vi "TCP Recieve Message.vi"(6 "Close on error":bool, 7 "Magic":u32=3737844653 format="%x", 8 "Error In":errorcluster, 11 "connection ID":refnum<k5>) -> (0 "Error Out":errorcluster, 1 "Valid":bool, 2 "Response":string, 3 "connection ID out":refnum<k5>)   [LabVIEW 2019]
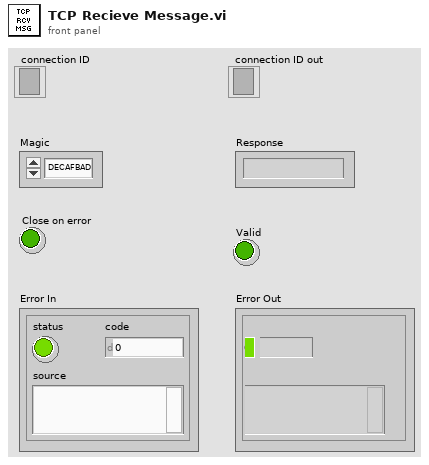
[diagram p1: front panel]
types:
  T1 = enum16{"big-endian, network order", "native, host order", "little-endian"}
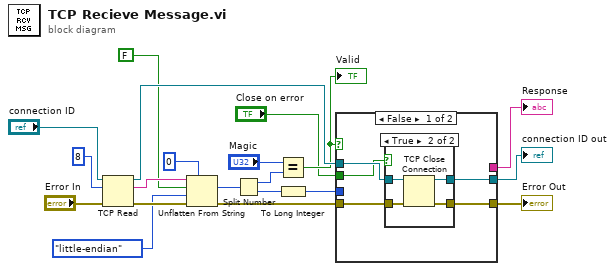
[diagram p0: block diagram]
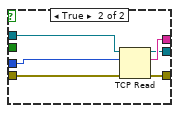
[diagram p3: hidden frame]
diagram:
  n1 = TCP Read(connection ID="connection ID", bytes to read=8, error in (no error)="Error In") -> (connection ID out=w14:refnum<k5>, data out=w5:string, error out=w7:errorcluster)  [unwired: 2 in]
  n2 = Unflatten From String(type=u64 0 ("x"), binary string=w5, data includes array or string size? (T)=FALSE, byte order (0:big-endian, network order)=T1."little-endian", error in (no error)=w7) -> (value=w1:u64, error out=w6:errorcluster)  [unwired: 1 out]
  n3 = Split Number(x=w1) -> (hi(x)=w17:u32, lo(x)=w15:u32)
  n4 = Equal?(x="Magic", y=w17) -> (x = y?=w9:bool)
  "Valid" <- w9
  n5 = To Long Integer(number=w15) -> (32bit integer=w13:i32)
  n6 = case shown="False" w9 {
    tunnel: w6 -> [w24 w37]
    tunnel: w13 -> [_ w36]
    tunnel: w14 -> [w25 w35]
    tunnel: [w23 w34] -> w12
    tunnel: [_ w33] -> w11
    tunnel: [w22 w32] -> w10
    tunnel: "Close on error" -> [w21 _]
    frame False {
      n7 = case shown="True" w21 {
        tunnel: w25 -> [w26 w31]
        tunnel: w24 -> [w27 w30]
        tunnel: [w27 w29] -> w23
        tunnel: [w26 w28] -> w22
        frame False {
        }
        frame True {
          n8 = TCP Close Connection(connection ID=w31, error in (no error)=w30) -> (connection ID out=w28:refnum<k5>, error out=w29:errorcluster)  [unwired: 1 in]
        }
      }
    }
    frame True {
      n9 = TCP Read(connection ID=w35, bytes to read=w36, error in (no error)=w37) -> (connection ID out=w32:refnum<k5>, data out=w33:string, error out=w34:errorcluster)  [unwired: 2 in]
    }
  }
  "Error Out" <- w12
  "Response" <- w11
  "connection ID out" <- w10
